vi "发送指令.vi"(8 "error in (no error)":errorcluster caption="错误输入（无错误）", 10 "指令":string, 11 "客户端 输入":refnum<class "客户端.lvclass">) -> (0 "error out":errorcluster caption="错误输出", 3 "客户端 输出":refnum<class "客户端.lvclass">)   [LabVIEW 2015, in "客户端.lvlib" / "客户端.lvclass"]
uses:
  <vilib>/Instr/_visa.llb/VISA Configure Serial Port (Instr).vi
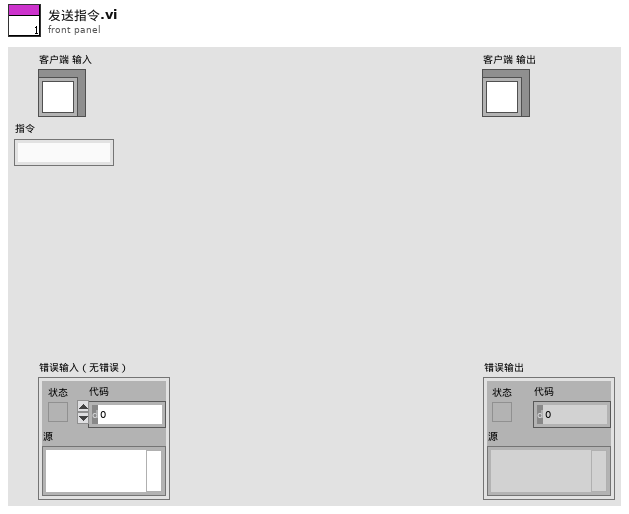
[diagram p1: front panel]
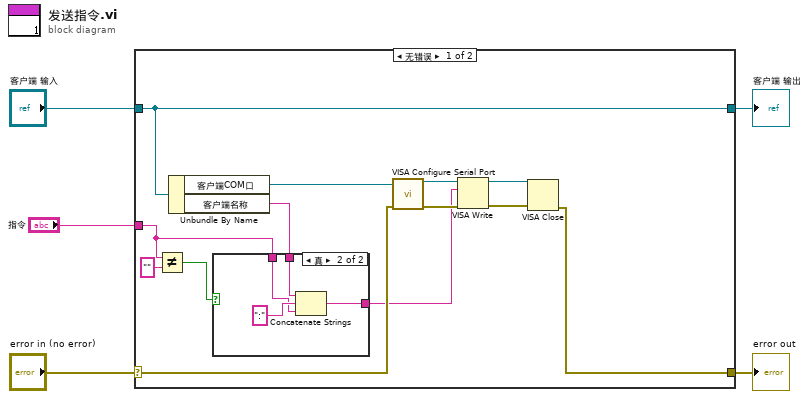
[diagram p0: block diagram]
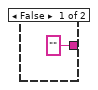
[diagram p2: hidden frame]
diagram:
  n1 = case shown="无错误" "error in (no error)" {
    selector: "error in (no error)" -> [w15 w25]
    tunnel: [w11 w25] -> w4
    tunnel: [w18 w24] -> w2
    tunnel: "客户端 输入" -> [w18 w24]
    tunnel: "指令" -> [w6 _]
    frame No Error {
      n2 = Not Equal?(x=w6, y="") -> (x != y?=w9:bool)
      n3 = Unbundle By Name(w18) -> ("客户端COM口"=w17:refnum<visa-resource-name>, "客户端名称"=w8:string)
      n4 = case shown="真" w9 {
        tunnel: w8 -> [_ w21]
        tunnel: ["" w22] -> w7
        tunnel: w6 -> [_ w20]
        frame False {
        }
        frame True {
          n5 = Concatenate Strings(w21, ":" ("字符串"), w20) -> (w22:string)
        }
      }
      n6 = call-poly "VISA Configure Serial Port"("VISA resource name"=w17, "error in (no error)"=w15) -> ("VISA resource name out"=w16:refnum<visa-resource-name>, "error out"=w14:errorcluster)  [unwired: 12 in]
      n7 = VISA Write(VISA resource name=w16, write buffer=w7, error in (no error)=w14) -> (VISA resource name out=w12:refnum<visa-resource-name>, error out=w13:errorcluster)  [unwired: 1 out]
      n8 = VISA Close(VISA resource name=w12, error in (no error)=w13) -> (error out=w11:errorcluster)
    }
    frame Error {
    }
  }
  "error out" <- w4
  "客户端 输出" <- w2
